vi "Rename Macro.vi"(8 "error in (no error)":errorcluster, 9 "Old Macro Name":string, 10 "New Macro Name":string, 11 "Motions in":refnum<class "Motions.lvclass">) -> (0 "error out":errorcluster, 2 "renamed successful":bool, 3 "Motions out":refnum<class "Motions.lvclass">)   [LabVIEW 2016, in "Hardware.lvlib" / "Motions.lvlib" / "Motions.lvclass"]
uses:
  <userlib>/Common Components/Hardware/Abstract System/Motions/Motions/Motions.lvclass
  <userlib>/Common Components/Hardware/Abstract System/Motions/Motions/Motions.lvclass/Motions.ctl
  <userlib>/Common Components/TriggerAction Q/TriggerAction Q/TriggerAction Q.lvclass
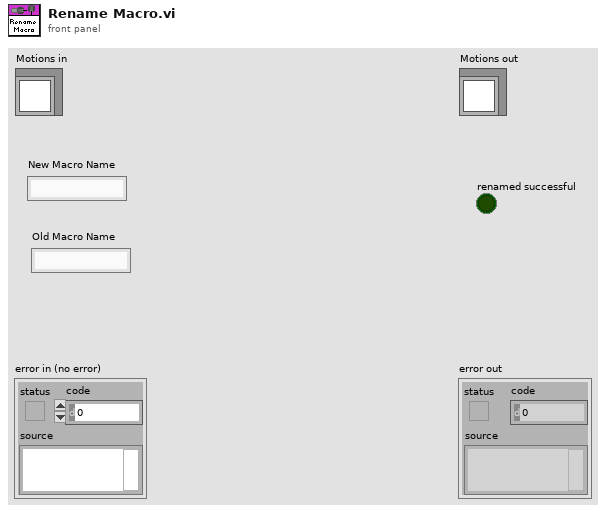
[diagram p1: front panel]
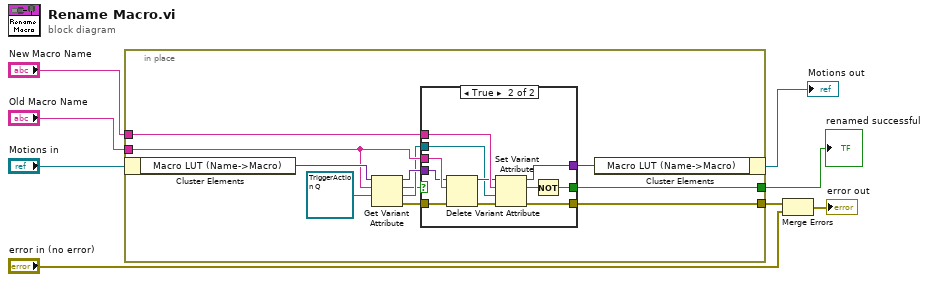
[diagram p0: block diagram]
diagram:
  n1 = in-place {
    in-place-border: "New Macro Name" -> [w17]
    in-place-border: [w16] -> w4
    in-place-border: [w9] -> w2
    in-place-border: "Old Macro Name" -> [w15]
    n2 = in-place-cluster #1("Motions in") -> ("Macro LUT (Name->Macro)"=w19:variant)
    n3 = Get Variant Attribute(Variant=w19, name=w15, default value (empty Variant)=refnum<class "TriggerAction Q.lvclass"> refnum ("TriggerAction Q.lvclass")) -> (duplicate Variant=w14:variant, found=w11:bool, value=w12:refnum<class "TriggerAction Q.lvclass">, error out=w10:errorcluster)  [unwired: 1 in]
    n4 = case shown="True" w11 {
      tunnel: [w20 w32] -> w18
      tunnel: w17 -> [_ w31]
      tunnel: [w21 w30] -> w16
      tunnel: w15 -> [_ w28]
      tunnel: w14 -> [w20 w27]
      tunnel: w12 -> [_ w26]
      tunnel: w10 -> [w21 w25]
      tunnel: [_ w22] -> w9
      frame False {
      }
      frame True {
        n5 = Delete Variant Attribute(4:w25, 6:w28, 7:w27) -> (0:w24:errorcluster, 3:w29:variant)  [unwired: 1 out]
        n6 = Set Variant Attribute(Variant=w29, name=w31, value=w26, error in=w24) -> (Variant out=w32:variant, replaced=w23:bool, error out=w30:errorcluster)
        n7 = Not(x=w23) -> (.not. x?=w22:bool)
      }
    }
    n8 = in-place-cluster #1("Macro LUT (Name->Macro)"=w18) -> (→"Motions out":refnum<class "Motions.lvclass">)
  }
  "renamed successful" <- w2
  n9 = Merge Errors(w4, "error in (no error)") -> (→"error out":errorcluster)
